vi "Read Child Actor Attributes.vi"(11 "Base Actor in":refnum<class "Base Actor.lvclass">) -> (2 "Child Actor Attributes":T1)   [LabVIEW 2020, in "jettl.lvlib" / "Base jettl Actor.lvlib" / "Base Actor.lvlib" / "Base Actor.lvclass"]
uses:
  Base Actor.lvclass
  Base Actor.lvclass/Base Actor.ctl
  Msg/Msg.lvclass
  Msg Input/Msg Input.lvclass
  Msg Output/Msg Output.lvclass
  Actor/Actor.lvclass
  Child Unified Actor.ctl
  jettl.lvlib
  Unified Actor.ctl
  Msg Set.ctl
  Unified Actor Relation.ctl
  Teller.ctl
  Msg.ctl
  Msgs.ctl
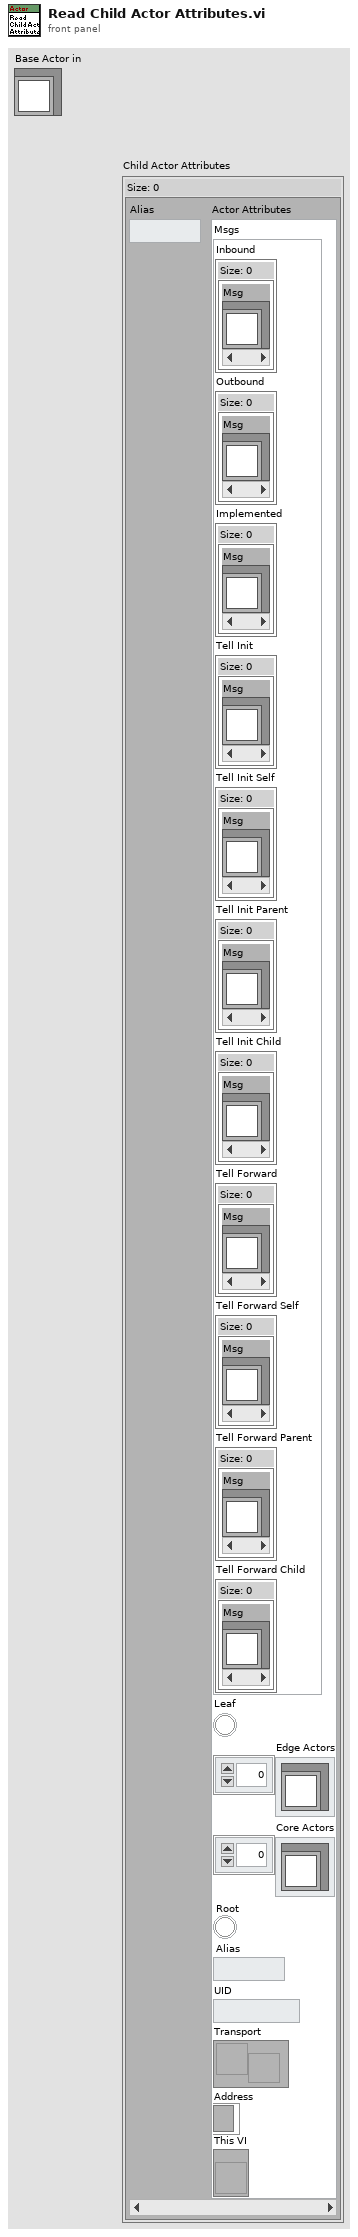
[diagram p1: front panel]
types:
  T1 = typedef "jettl.lvlib/Child Unified Actor.ctl" = map{string, T2}
  T2 = typedef "jettl.lvlib/Unified Actor.ctl" = cluster{"Msgs":T3, "Leaf":bool, "Edge Actors":refnum<class "Actor.lvclass">[], "Core Actors":refnum<class "Actor.lvclass">[], "Root":bool, "Alias":string, "UID":i32, "Transport":refnum<user-event>, "Address":refnum<event-registration>, "This VI":refnum<vi>}
  T3 = typedef "jettl.lvlib/Msgs.ctl" = cluster{"Inbound":T4, "Outbound":T4, "Implemented":T4, "Tell Init":T4, "Tell Init Self":T4, "Tell Init Parent":T4, "Tell Init Child":T4, "Tell Forward":T4, "Tell Forward Self":T4, "Tell Forward Parent":T4, "Tell Forward Child":T4}
  T4 = typedef "jettl.lvlib/Msg Set.ctl" = set{refnum<class "Msg.lvclass">}
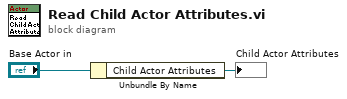
[diagram p0: block diagram]
diagram:
  n1 = Unbundle By Name("Base Actor in") -> ("Child Actor Attributes"=→"Child Actor Attributes":refnum<data-value>)
